vi "PrimeTXT_parse.vi"() -> (12 "file path (dialog if empty)":path=path "C:/Users/MUSE_V2/Desktop/CLIO/DensityPumpSettings.txt", 14 "Strokes_solvent":i32, 15 "Strokes_air":i32, 16 "Strokes_prime":i32, 17 "Iterations":i32, 18 "RPM_air":i32, 19 "RPM_prime":i32)   [LabVIEW 2019]
uses:
  <vilib>/Utility/file.llb/Read Delimited Spreadsheet (I64).vi
panel:
  out "all rows":i32[][](array[numeric])
  # "ady changed strokes_prime: 50 > 95 (1/12/2021)"
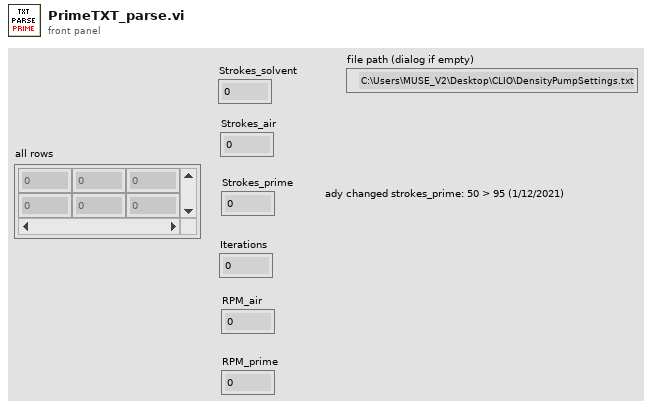
[diagram p1: front panel]
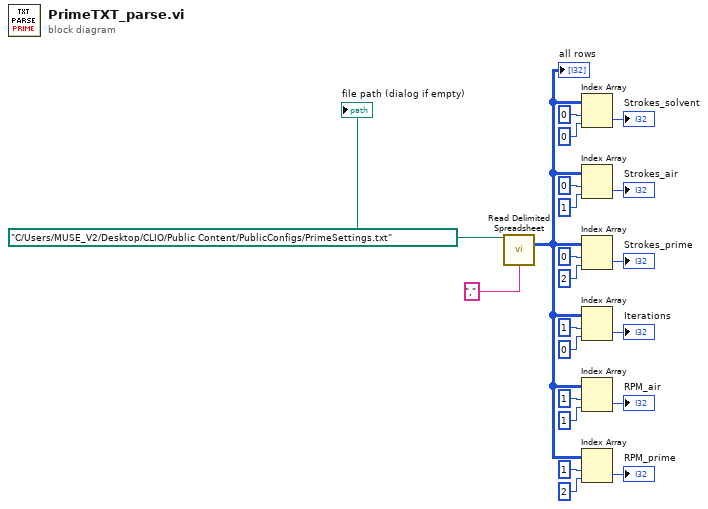
[diagram p0: block diagram]
diagram:
  w21 = path "C:/Users/MUSE_V2/Desktop/CLIO/Public Content/PublicConfigs/PrimeSettings.txt" ("file path (dialog if empty)")
  n1 = call-poly <vilib>:"Read Delimited Spreadsheet.vi"("file path (dialog if empty)"=w21, "delimiter (\\t)"="," ("delimiter (\\t)")) -> ("all rows"=w1:i64[][])  [unwired: 8 in, 5 out]
  "all rows" <- w1
  n2 = Index Array(array=w1, index (row)=0, index (col)=0 ("disabled index (col)")) -> (element=→"Strokes_solvent":i64)
  n3 = Index Array(array=w1, index (row)=0, index (col)=1 ("disabled index (col)")) -> (element=→"Strokes_air":i64)
  n4 = Index Array(array=w1, index (row)=0, index (col)=2 ("disabled index (col)")) -> (element=→"Strokes_prime":i64)
  n5 = Index Array(array=w1, index (row)=1, index (col)=0 ("disabled index (col)")) -> (element=→"Iterations":i64)
  n6 = Index Array(array=w1, index (row)=1, index (col)=1 ("disabled index (col)")) -> (element=→"RPM_air":i64)
  n7 = Index Array(array=w1, index (row)=1, index (col)=2 ("disabled index (col)")) -> (element=→"RPM_prime":i64)
  "file path (dialog if empty)" <- w21
